vi "Solve2.vi"(8 "Error In":errorcluster, 11 "object in":refnum<class "2021_10.lvclass">) -> (0 "Error Out":errorcluster, 2 "Result":u64, 3 "object out":refnum<class "2021_10.lvclass">)   [LabVIEW 2020, in "2021_10.lvclass"]
uses:
  2021_10.lvclass
  2021_10.lvclass/2021_10.ctl
  <vilib>/Analysis/NI_AALBase.lvlib
panel:
  out "Array":string[](array[string])
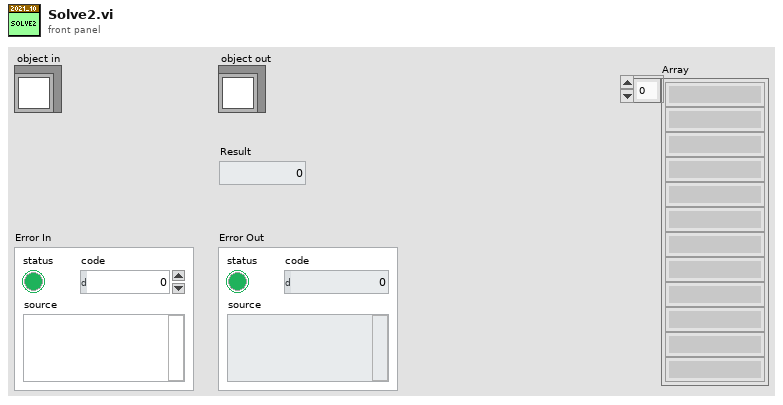
[diagram p1: front panel]
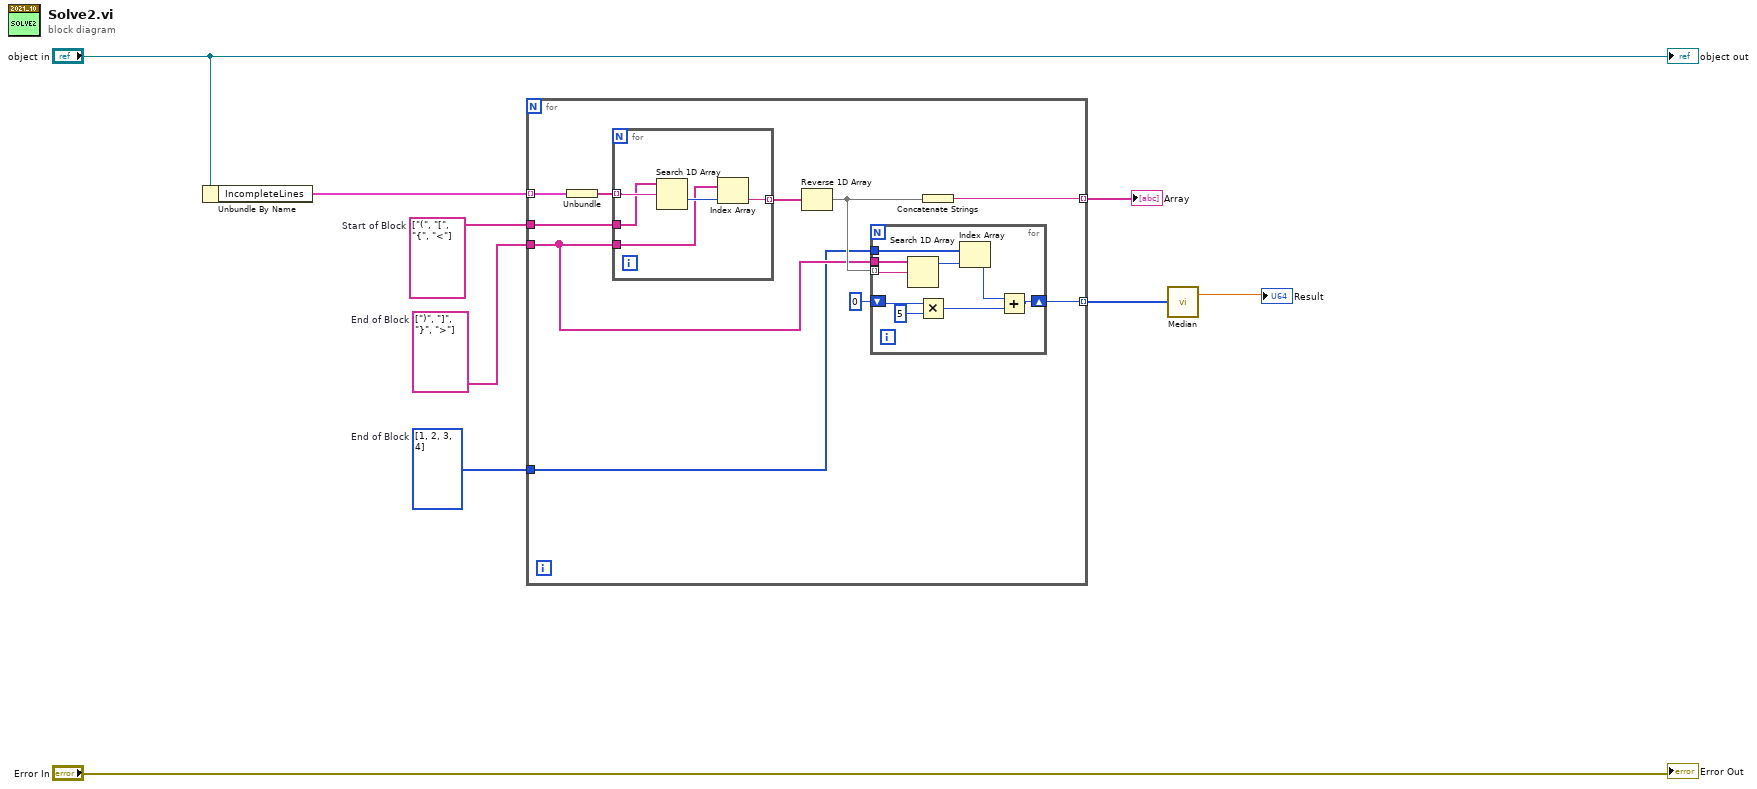
[diagram p0: block diagram]
diagram:
  w3 = u64[] [1, 2, 3, 4]  # End of Block
  w5 = string[] [")", "]", "}", ">"]  # End of Block
  w6 = string[] ["(", "[", "{", "<"]  # Start of Block
  n1 = Unbundle By Name("object in") -> ("IncompleteLines"=w7:cluster{string[]}[])
  n2 = for {
    tunnel: w7 -> [w19] mode=indexing
    tunnel: w6 -> [w17]
    tunnel: w5 -> [w13]
    tunnel: [w16] -> w4 mode=indexing
    tunnel: w3 -> [w12]
    tunnel: [w10] -> w2 mode=indexing
    n3 = Unbundle(w19) -> (w18:string[])
    n4 = for {
      tunnel: w18 -> [w33] mode=indexing
      tunnel: w17 -> [w32]
      tunnel: w13 -> [w30]
      tunnel: [w29] -> w15 mode=indexing
      n5 = Search 1D Array(1D array=w32, element=w33) -> (index of element=w31:i32)  [unwired: 1 in]
      n6 = Index Array(array=w30, index=w31) -> (element=w29:string)
    }
    n7 = Reverse 1D Array(array=w15) -> (reversed array=w14:string[])
    n8 = for {
      tunnel: w14 -> [w26] mode=indexing
      shift-right: [w20] -> w10
      shift-left: u64 0 -> [w28]
      tunnel: w13 -> [w25]
      tunnel: w12 -> [w23]
      n9 = Search 1D Array(1D array=w25, element=w26) -> (index of element=w24:i32)  [unwired: 1 in]
      n10 = Multiply(x=w28, y=u64 5) -> (x*y=w22:u64)
      n11 = Index Array(array=w23, index=w24) -> (element=w21:u64)
      n12 = Add(x=w21, y=w22) -> (x+y=w20:u64)
    }
    n13 = Concatenate Strings(w14) -> (w16:string)
  }
  "Array" <- w4
  n14 = call <vilib>:"Median.vi"("X"=w2) -> ("median"=→"Result":dbl)  [unwired: 1 out]
  "Error Out" <- "Error In"
  "object out" <- "object in"
